vi "Read_Field.vi"() -> ()   [LabVIEW 2016]
uses:
  Instrument_Setup.vi
panel:
  out "error in (no error) 2":errorcluster
  in  "error in (no error)":errorcluster
  out "Numeric 2":dbl format="%#_13g"
  out "Numeric":dbl format="%#_13g"
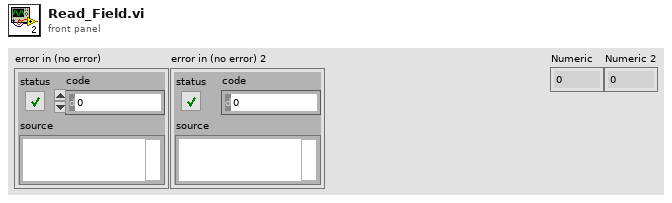
[diagram p1: front panel]
types:
  T1 = cluster{"GPIB address":i16, "GPIB bus":i16, "connection ID":refnum<k5>, "IP":string, "Active Comm Interface":u16, "Serial Port":refnum<visa-resource-name>, "Programmer Type":u16}
  T2 = cluster{"error":bool, "code":i32, "source":string}
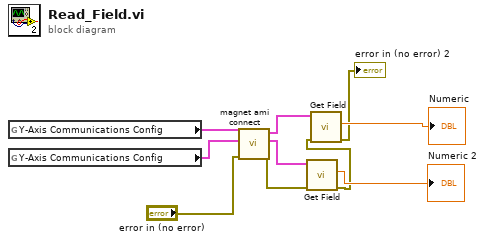
[diagram p0: block diagram]
diagram:
  n1 = global read "Instrument_Setup.vi" "Y-Axis Communications Config"() -> (w8:T1)
  n2 = global read "Instrument_Setup.vi" "Y-Axis Communications Config"() -> (w7:T1)
  n3 = call "magnet ami connect.vi"("error in (no error)"="error in (no error)", "Z-Axis Communications Config"=w7, "Y-Axis Communications Config"=w8) -> ("error out"=w4:errorcluster, "Z-Axis Communications Config Out"=w5:T1, "Y-Axis Communications Config Out"=w6:T1)  [unwired: 6 in]
  n4 = call "Get Field.vi"("Z-Axis Communications Config"=w5, "error in"=w4) -> ("Field(T)"=→"Numeric 2":dbl, "error out"=w3:T2)  [unwired: 4 in, 1 out]
  n5 = call "Get Field.vi"("Z-Axis Communications Config"=w6, "error in"=w3) -> ("Field(T)"=→"Numeric":dbl, "error out"=→"error in (no error) 2":T2)  [unwired: 4 in, 1 out]
